vi "Run VI UI.vi"() -> ()   [LabVIEW 2014, in "Run VI Node.lvclass"]
uses:
  Run VI Node.lvclass
  <vilib>/ni/Configuration Framework/Node/NodeRef.ctl
  <vilib>/ni/Configuration Framework/Node/NISE_CEF_Node.lvclass
  <vilib>/ni/AMC/Message Queue.ctl
  <vilib>/ni/AMC/Message.ctl
  <vilib>/ni/Tools/Keyed Array/KeyedArray.ctl
  <vilib>/ni/Configuration Framework/Node/UserEventRef.ctl
  <vilib>/ni/Configuration Framework/Controls/EventCluster.ctl
  Run VI Node.lvclass/Run VI Node.ctl
  Classes/Build Job/Build Job.lvclass/Build Job.ctl
  <vilib>/ni/AMC/Create Single Message.vi
  <vilib>/ni/AMC/Update Message Routing Info.vi
  <vilib>/ni/AMC/Send Message.vi
  <vilib>/ni/AMC/AMC.lvlib
  Classes/Build Job/Build Job.lvclass
  <vilib>/ni/Tools/Keyed Array/Tools_KeyedArray.lvlib
  <vilib>/ni/Configuration Framework/NISE_CEF_TreeControl.lvlib
panel:
  in  "Description":string="brandyn.adderley@ni.com"
  in  "Wait Until Done?":bool
  in  "VI Path":path=path "C:/Projects/LabVIEW Continuous Integration/LabVIEW Continuous Integration.lvproj"
  in  "user event":T1
  in  "main queue":T2
  in  "node ref":T3
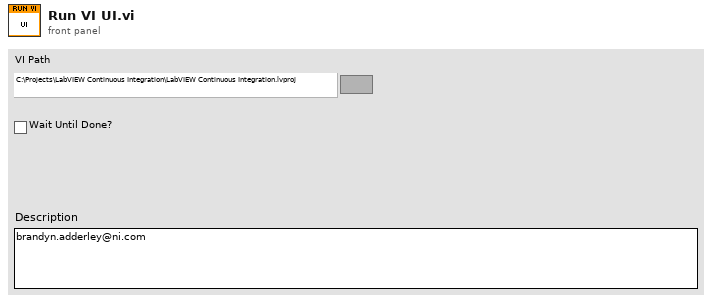
[diagram p1: front panel]
types:
  T1 = typedef "NISE_CEF_Node.lvclass/UserEventRef.ctl" = refnum<user-event>
  T2 = typedef "AMC.lvlib/Message Queue.ctl" = refnum<queue>
  T3 = typedef "NISE_CEF_Node.lvclass/NodeRef.ctl" = refnum<data-value>
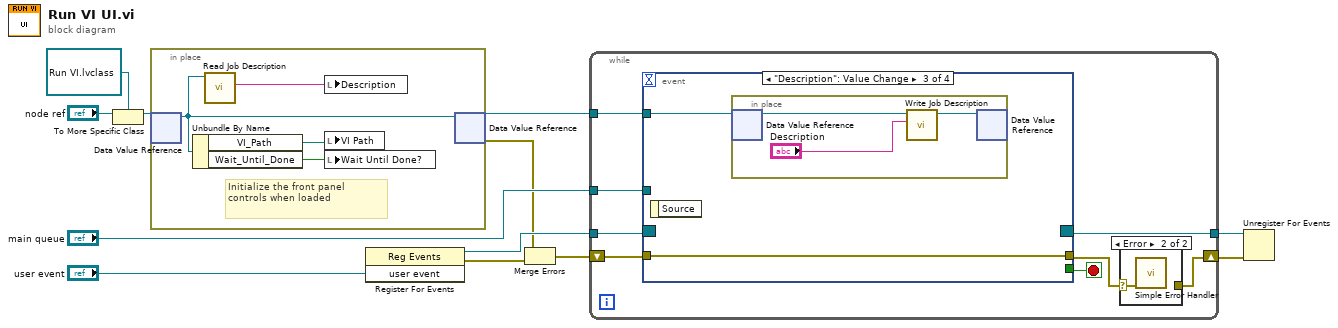
[diagram p0: block diagram]
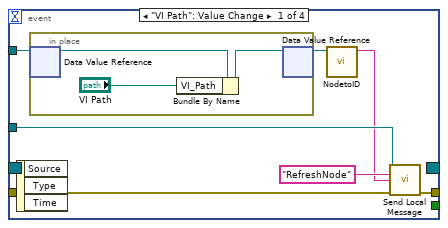
[diagram p3: hidden frame]
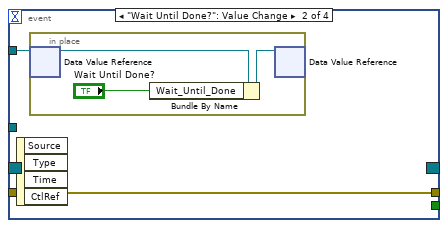
[diagram p4: hidden frame]
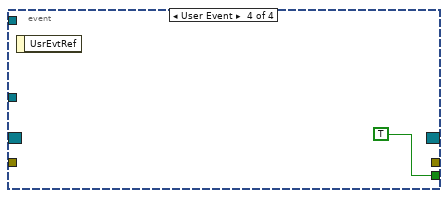
[diagram p5: hidden frame]
diagram:
  n1 = To More Specific Class(target class=refnum<data-value> refnum ("data value reference"), reference="node ref") -> (specific class reference=w5:refnum<data-value>)  [unwired: 1 in, 1 out]
  n2 = in-place {
    # "Initialize the front panel controls when loaded"
    n3 = in-place-dvr #1(w5) -> (w13:refnum<class "Run VI Node.lvclass">)  [unwired: 1 out]
    n4 = Unbundle By Name(w13) -> ("VI_Path"=w16:path, "Wait_Until_Done"=w15:bool)
    n5 = call-dynamic "Read Job Description.vi"("Build Job in"=w13) -> ("Job Description"=w14:string)  [unwired: 10 in]
    n6 = local write "Description"(w14) -> ()
    n7 = local write "VI Path"(w16) -> ()
    n8 = local write "Wait Until Done?"(w15) -> ()
    n9 = in-place-dvr #1(w13) -> (w12:refnum<data-value>, w2:errorcluster)
  }
  n10 = register-events("user event") -> (reference out=w9:refnum<event-registration>, error out=w3:errorcluster)  [unwired: 2 in]
  n11 = Merge Errors(w2, w3) -> (w1:errorcluster)
  n12 = while {
    tunnel: w12 -> [w24]
    tunnel: "main queue" -> [w23]
    tunnel: w9 -> [w22]
    tunnel: [w21] -> w8
    shift-right: [w17] -> w7
    shift-left: w1 -> [w20]
    stop <- w19 stop-if-true
    n13 = event shown="[2] \"Description\": Value Change" {
      selector: w22 -> [_ _ _ _]
      dyn-events: [_ _ _ _] -> w21
      timeout: _ -> [_ _ _ _]
      tunnel: w24 -> [w31 w38 w43 _]
      tunnel: w23 -> [w32 _ _ _]
      tunnel: [_ _ _ TRUE] -> w19
      tunnel: [w29 w37 w42 _] -> w18
      tunnel: w20 -> [w28 w37 w42 _]
      event "VI Path": Value Change {
        n14 = event-data() -> ()  [unwired: 1 in, 3 out]
        n15 = in-place {
          n16 = in-place-dvr #2(w31) -> (w36:refnum<class "Run VI Node.lvclass">)  [unwired: 1 out]
          n17 = Bundle By Name(cluster=w36, "VI_Path"="VI Path") -> (w35:refnum<class "Run VI Node.lvclass">)
          n18 = in-place-dvr #2(w35) -> (w27:refnum<data-value>)  [unwired: 1 out]
        }
        n19 = call <vilib>:"NodetoID.vi"("node ref"=w27) -> ("ID"=w30:string)  [unwired: 9 in, 1 out]
        n20 = call <vilib>:"Send Local Message.vi"("message queue in"=w32, "message name"="RefreshNode" ("Message Name"), "message value"=w30, "error in"=w28) -> ("error out"=w29:errorcluster)  [unwired: 9 in, 2 out]
      }
      event "Wait Until Done?": Value Change {
        n21 = event-data() -> ()  [unwired: 1 in, 4 out]
        n22 = in-place {
          n23 = in-place-dvr #3(w38) -> (w41:refnum<class "Run VI Node.lvclass">)  [unwired: 1 out]
          n24 = Bundle By Name(cluster=w41, "Wait_Until_Done"="Wait Until Done?") -> (w40:refnum<class "Run VI Node.lvclass">)
          n25 = in-place-dvr #3(w40) -> ()  [unwired: 2 out]
        }
      }
      event "Description": Value Change {
        n26 = event-data() -> ()  [unwired: 1 in, 1 out]
        n27 = in-place {
          n28 = in-place-dvr #4(w43) -> (w46:refnum<class "Run VI Node.lvclass">)  [unwired: 1 out]
          n29 = call "Write Job Description.vi"("Job Description"="Description", "Build Job in"=w46) -> ("Build Job out"=w45:refnum<class "Run VI Node.lvclass">)  [unwired: 9 in]
          n30 = in-place-dvr #4(w45) -> ()  [unwired: 2 out]
        }
      }
      event User Event {
        n31 = event-data() -> ()  [unwired: 1 in, 1 out]
      }
    }
    n32 = case shown="Error" w18 {
      selector: w18 -> [w25 w26]
      tunnel: [w25 _] -> w17
      frame No Error {
      }
      frame Error {
        n33 = call <vilib>:"Simple Error Handler.vi"("error in (no error)"=w26) -> ()  [unwired: 4 in, 5 out]
      }
    }
  }
  n34 = Unregister For Events(event registration refnum=w8, error in=w7) -> ()  [unwired: 1 out]
